vi "program.vi"() -> ()   [LabVIEW 2015]
panel:
  in  "Tab Control":enum32{"control", "diagnostics"}(tab)
  in  "Program":T1(array[cluster])=[{"Tstart"=95.0, "Tstop"=95.0, "rate(C/min)"=0.0, "time(min)"=5.0}, {"Tstart"=95.0, "Tstop"=90.0, "rate(C/min)"=240.0, "time(min)"=0.0}, {"Tstart"=90.0, "Tstop"=76.0, "rate(C/min)"=0.2, "time(min)"=0.0}, {"Tstart"=76.0, "Tstop"=26.0, "rate(C/min)"=0.067, "time(min)"=0.0}, {"Tstart"=25.0, "Tstop"=25.0, "rate(C/min)"=0.0, "time(min)"=30.0}] {"Tstop" min=20.0 max=100.0; "Tstart" min=20.0 max=100.0}
  out "XY Graph":cluster{dbl[], dbl[]}[](graph)
  out "temperature":dbl format="%.1f"
  in  "run":bool
  in  "abort":bool
  out "state":T2(ring)
  out "setpoint":dbl format="%.1f"
  in  "tolerance":dbl=1.0 format="%.2f"
  out "?":string
  out "concatenated string":string
  in  "dt(min)":dbl=1.0
  out "ptrace":cluster{dbl[], dbl[]}
  # "Instructions:  \n    1) Edit the program before starting the  VI\n    2) After starting, Hit Run or Abort as needed."
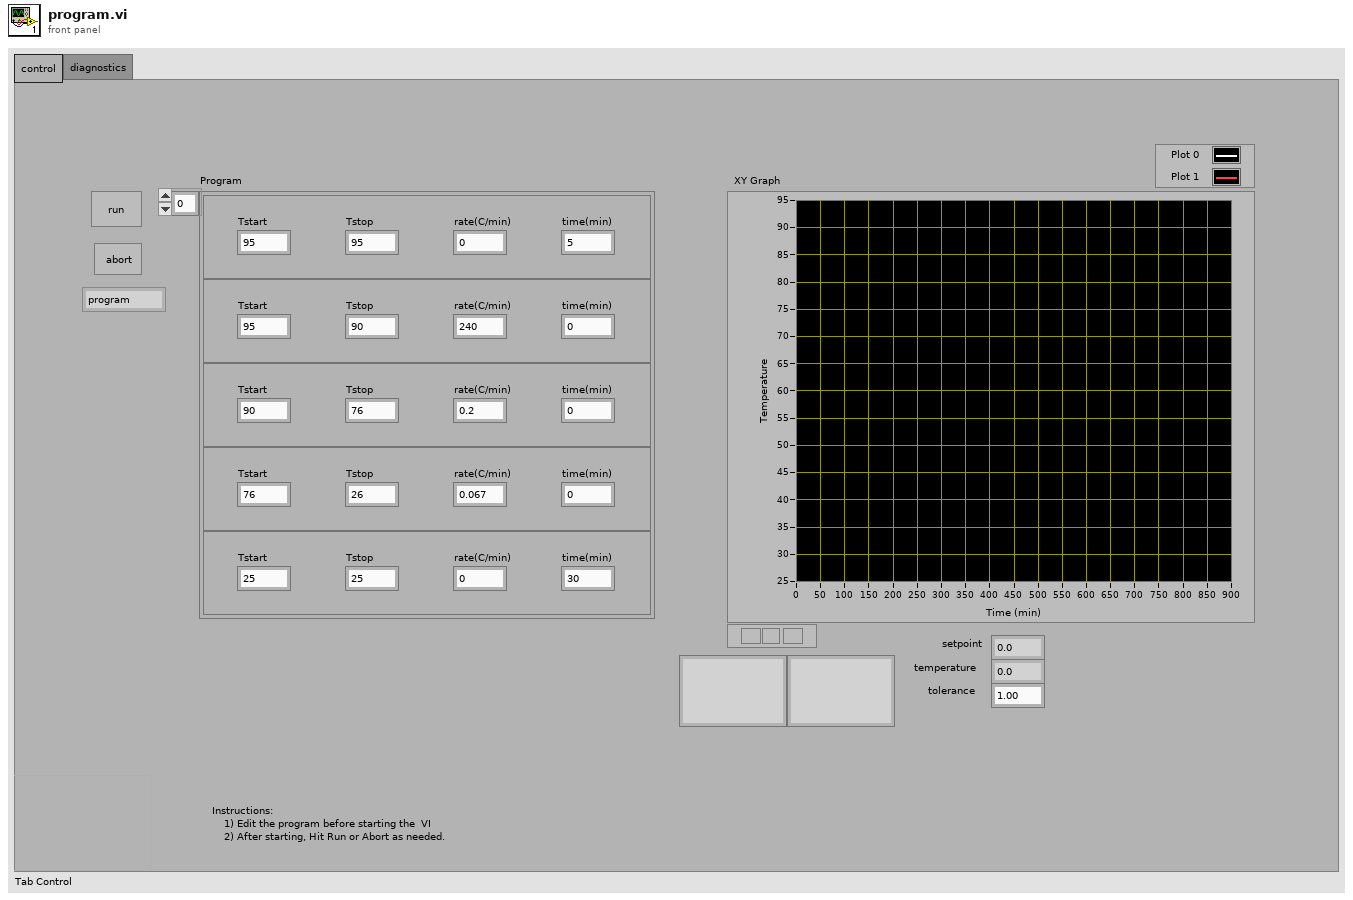
[diagram p1: front panel]
types:
  T1 = cluster{"Tstart":dbl, "Tstop":dbl, "rate(C/min)":dbl, "time(min)":dbl}[]
  T2 = enum16{"program", "init", "follow", "aborting", "quit"}
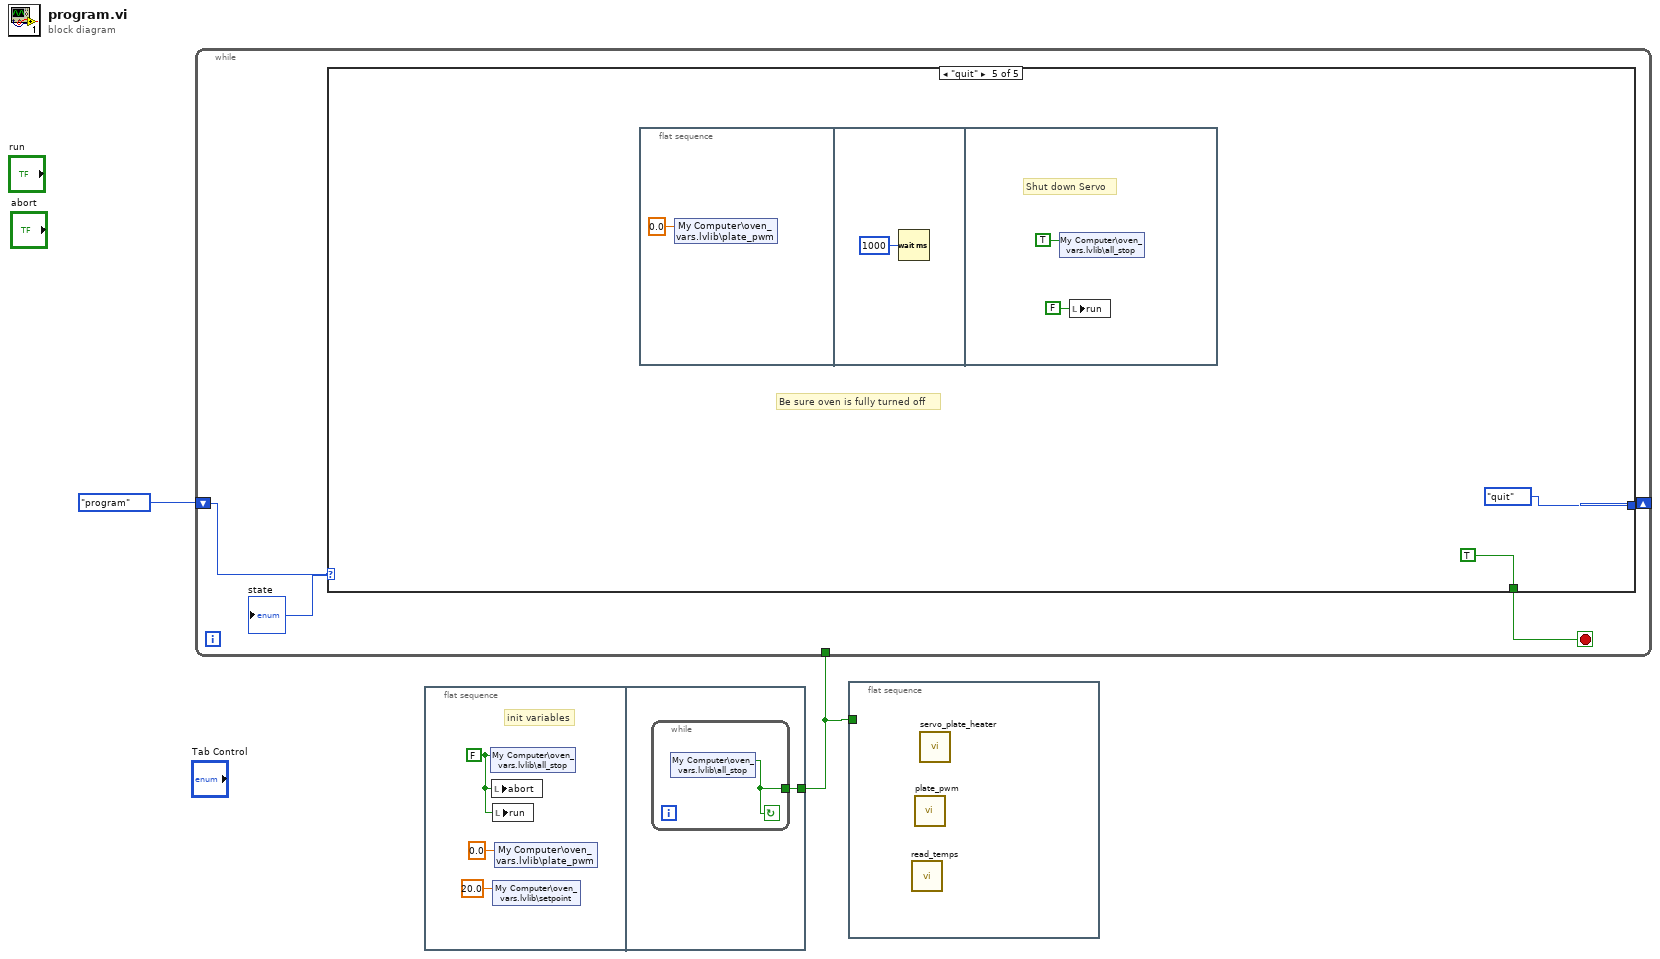
[diagram p0: block diagram]
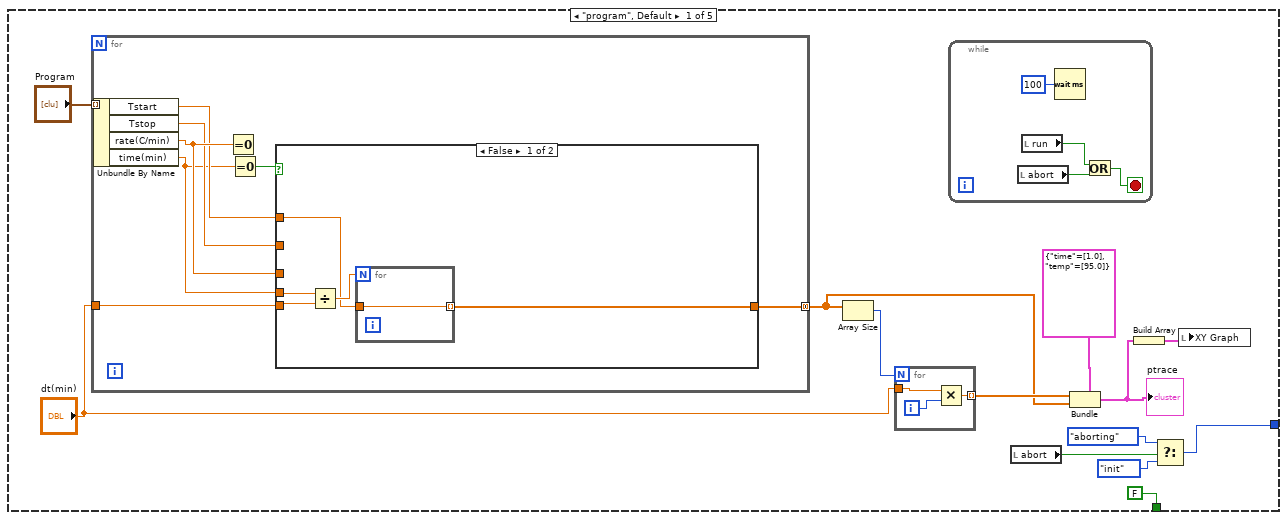
[diagram p2: hidden frame]
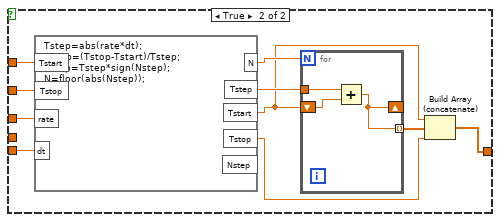
[diagram p3: hidden frame]
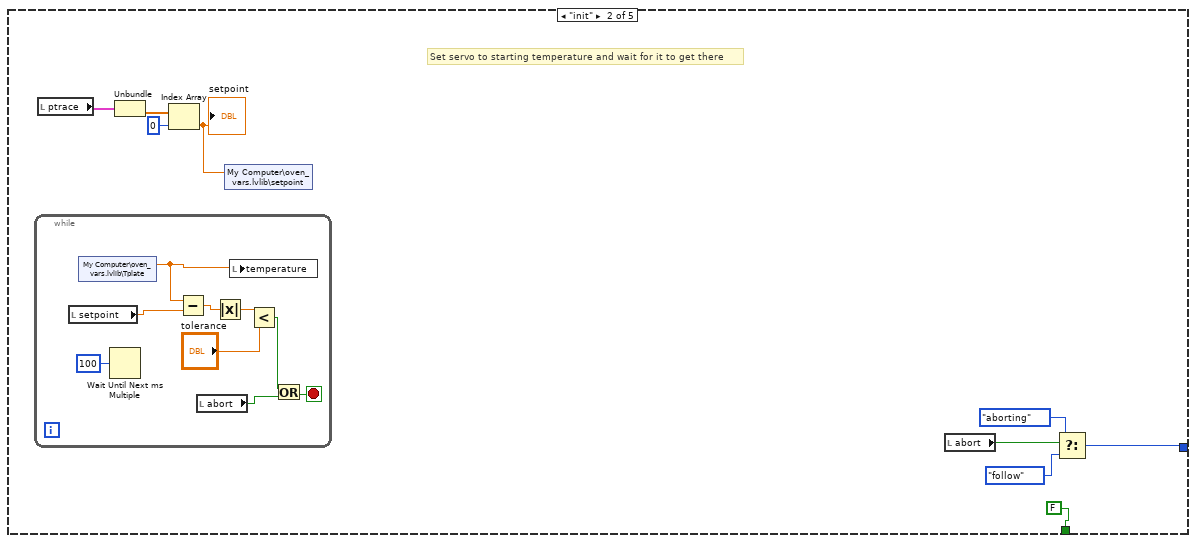
[diagram p4: hidden frame]
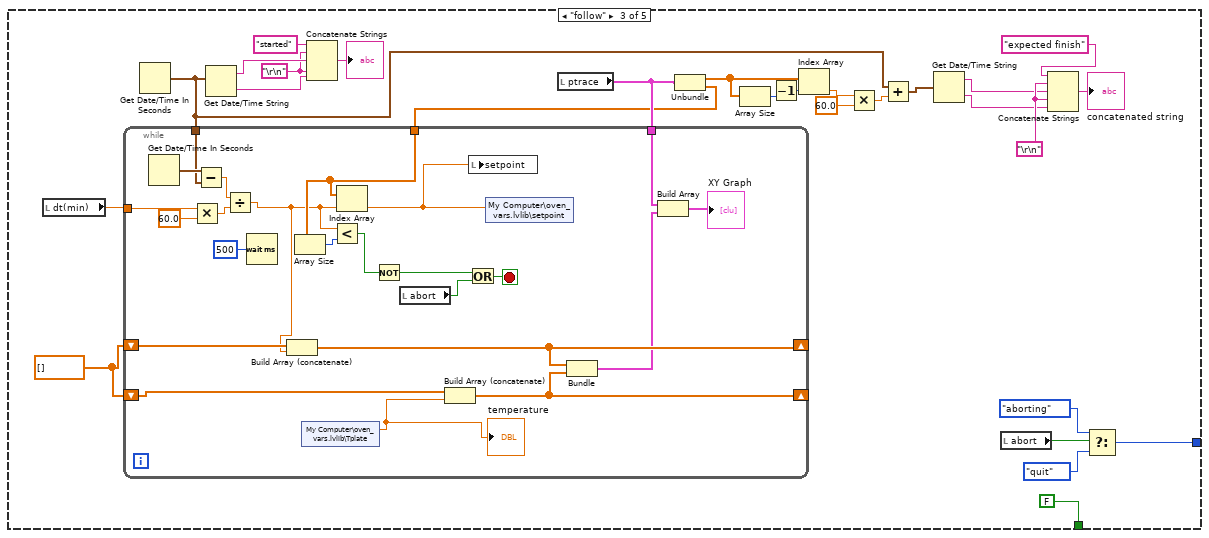
[diagram p5: hidden frame]
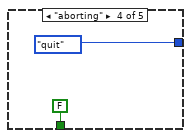
[diagram p6: hidden frame]
diagram:
  n1 = while {
    shift-right: [w5] -> _
    shift-left: T2."program" ("state") -> [w3]
    tunnel: w1 -> [_]
    stop <- w4 stop-if-true
    n2 = case shown="\"quit\"" w3 {
      tunnel: [w11 w57 w93 T2."quit" ("state") T2."quit" ("state")] -> w5
      tunnel: [FALSE FALSE FALSE FALSE TRUE] -> w4
      frame "program", Default {
        n3 = for {
          tunnel: "Program" -> [w33] mode=indexing
          tunnel: [w27] -> w14 mode=concatenating
          tunnel: "dt(min)" -> [w26]
          n4 = Unbundle By Name(w33) -> ("Tstart"=w31:dbl, "Tstop"=w30:dbl, "rate(C/min)"=w32:dbl, "time(min)"=w28:dbl)
          n5 = Equal To 0?(x=w32) -> ()  [unwired: 1 out]
          n6 = Equal To 0?(x=w28) -> (x = 0?=w29:bool)
          n7 = case shown="False" w29 {
            tunnel: w26 -> [w37 w49]
            tunnel: w32 -> [_ w48]
            tunnel: w31 -> [w35 w47]
            tunnel: w30 -> [_ w46]
            tunnel: w28 -> [w38 _]
            tunnel: [w34 w40] -> w27
            frame False {
              n8 = Divide(x=w38, y=w37) -> (x/y=w36:dbl)
              n9 = for {
                N: w36 -> [_]
                tunnel: w35 -> [w39]
                tunnel: [w39] -> w34 mode=indexing
              }
            }
            frame True {
              n10 = formula code="Tstep=abs(rate*dt);\nNstep=(Tstop-Tstart)/Tstep;\nTstep=Tstep*sign(Nstep);\nN=floor(abs(Nstep));"("Tstart"=w47, "Tstop"=w46, "rate"=w48, "dt"=w49) -> ("N"=w45:dbl, "Tstep"=w44:dbl, "Tstart"=w41:dbl, "Tstop"=w42:dbl)  [unwired: 1 out]
              n11 = for {
                N: w45 -> [_]
                shift-right: [w50] -> _
                shift-left: w41 -> [w52]
                tunnel: w44 -> [w51]
                tunnel: [w50] -> w43 mode=indexing
                n12 = Add(x=w51, y=w52) -> (x+y=w50:dbl)
              }
              n13 = Build Array (concatenate)(w41, w43, w42) -> (w40:dbl[])
            }
          }
        }
        n14 = Array Size(array=w14) -> (size(s)=w17:i32)
        n15 = for {
          N: w17 -> [_]
          tunnel: "dt(min)" -> [w24]
          tunnel: [w23] -> w16 mode=indexing
          i -> [w25]
          n16 = Multiply(x=w24, y=w25) -> (x*y=w23:dbl)
        }
        n17 = while {
          stop <- w22 stop-if-true
          n18 = local read "abort"() -> (w21:bool)
          n19 = local read "run"() -> (w20:bool)
          n20 = Wait (ms)(milliseconds to wait=u32 100) -> ()  [unwired: 1 out]
          n21 = Or(x=w20, y=w21) -> (x .or. y?=w22:bool)
        }
        n22 = local read "abort"() -> (w10:bool)
        n23 = Bundle(cluster=cluster{"time":dbl[], "temp":dbl[]} {"time"=[1.0], "temp"=[95.0]}, "time"=w16, "temp"=w14) -> (w6:cluster{"time":dbl[], "temp":dbl[]})
        "ptrace" <- w6
        n24 = Build Array(w6) -> (w7:cluster{"time":dbl[], "temp":dbl[]}[])
        n25 = Select(t=T2."aborting" ("state"), s=w10, f=T2."init" ("state")) -> (s? t:f=w11:T2)
        n26 = local write "XY Graph"(w7) -> ()
      }
      frame "init" {
        # "Set servo to starting temperature and wait for it to get there"
        n27 = while {
          stop <- w64 stop-if-true
          n28 = local read "setpoint"() -> (w70:dbl)
          n29 = shared-variable "My Computer\\oven_vars.lvlib\\Tplate"() -> (w62:dbl)  [unwired: 1 in, 1 out]
          n30 = Wait Until Next ms Multiple(millisecond multiple=u32 100) -> ()  [unwired: 1 out]
          n31 = Subtract(x=w62, y=w70) -> (x-y=w69:dbl)
          n32 = local read "abort"() -> (w63:bool)
          n33 = Absolute Value(x=w69) -> (abs(x)=w68:dbl)
          n34 = local write "temperature"(w62) -> ()
          n35 = Less?(x=w68, y="tolerance") -> (x < y?=w66:bool)
          n36 = Or(x=w66, y=w63) -> (x .or. y?=w64:bool)
        }
        n37 = local read "ptrace"() -> (w61:cluster{dbl[], dbl[]})
        n38 = Unbundle(w61) -> (w60:dbl[])  [unwired: 1 out]
        n39 = Index Array(array=w60, index=0) -> (element=w58:dbl)
        "setpoint" <- w58
        n40 = shared-variable "My Computer\\oven_vars.lvlib\\setpoint"(w58) -> ()  [unwired: 1 in, 1 out]
        n41 = local read "abort"() -> (w56:bool)
        n42 = Select(t=T2."aborting" ("state"), s=w56, f=T2."follow" ("state")) -> (s? t:f=w57:T2)
      }
      frame "follow" {
        w74 = "\r\n"
        w85 = "\r\n"
        w97 = dbl[] []
        n43 = local read "dt(min)"() -> (w94:dbl)
        n44 = Get Date/Time In Seconds() -> (seconds since 1Jan1904=w77:timestamp)
        n45 = Get Date/Time String(seconds (now)=w77) -> (date string=w87:string, time string=w86:string)  [unwired: 2 in]
        n46 = Concatenate Strings("started" ("string"), w85, w87, w85, w86) -> (→"?":string)
        n47 = local read "ptrace"() -> (w96:cluster{dbl[], dbl[]})
        n48 = Unbundle(w96) -> (w82:dbl[], w95:dbl[])
        n49 = while {
          tunnel: w77 -> [w119]
          tunnel: w94 -> [w115]
          tunnel: w95 -> [w104]
          shift-right: [w111] -> _
          shift-left: w97 -> [w113]
          shift-right: [w110] -> _
          shift-left: w97 -> [w112]
          tunnel: w96 -> [w108]
          stop <- w106 stop-if-true
          n50 = Get Date/Time In Seconds() -> (seconds since 1Jan1904=w120:timestamp)
          n51 = Multiply(x=w115, y=60.0) -> (x*y=w116:dbl)
          n52 = Subtract(x=w120, y=w119) -> (x-y=w117:dbl)
          n53 = Divide(x=w117, y=w116) -> (x/y=w102:dbl)
          n54 = Wait (ms)(milliseconds to wait=u32 500) -> ()  [unwired: 1 out]
          n55 = Build Array (concatenate)(w113, w102) -> (w111:dbl[])
          n56 = Array Size(array=w104) -> (size(s)=w103:i32)
          n57 = shared-variable "My Computer\\oven_vars.lvlib\\Tplate"() -> (w99:dbl)  [unwired: 1 in, 1 out]
          "temperature" <- w99
          n58 = Less?(x=w102, y=w103) -> (x < y?=w101:bool)
          n59 = Index Array(array=w104, index=w102) -> (element=w100:dbl)
          n60 = Not(x=w101) -> (.not. x?=w98:bool)
          n61 = local read "abort"() -> (w105:bool)
          n62 = Build Array (concatenate)(w112, w99) -> (w110:dbl[])
          n63 = Or(x=w98, y=w105) -> (x .or. y?=w106:bool)
          n64 = local write "setpoint"(w100) -> ()
          n65 = shared-variable "My Computer\\oven_vars.lvlib\\setpoint"(w100) -> ()  [unwired: 1 in, 1 out]
          n66 = Bundle(w111, w110) -> (w109:cluster{dbl[], dbl[]})  [unwired: 1 in]
          n67 = Build Array(w108, w109) -> (→"XY Graph":cluster{dbl[], dbl[]}[])
        }
        n68 = Array Size(array=w82) -> (size(s)=w83:i32)
        n69 = Decrement(x=w83) -> (x-1=w81:i32)
        n70 = Index Array(array=w82, index=w81) -> (element=w80:dbl)
        n71 = Multiply(x=w80, y=60.0) -> (x*y=w78:dbl)
        n72 = Add(x=w77, y=w78) -> (x+y=w76:timestamp)
        n73 = Get Date/Time String(seconds (now)=w76) -> (date string=w73:string, time string=w71:string)  [unwired: 2 in]
        n74 = local read "abort"() -> (w92:bool)
        n75 = Concatenate Strings("expected finish", w74, w73, w74, w71) -> (→"concatenated string":string)
        n76 = Select(t=T2."aborting" ("state"), s=w92, f=T2."quit" ("state")) -> (s? t:f=w93:T2)
      }
      frame "aborting" {
      }
      frame "quit" {
        # "Be sure oven is fully turned off"
        n77 = flat-sequence {
          frame #0 {
            n78 = shared-variable "My Computer\\oven_vars.lvlib\\plate_pwm"(0.0 ("plate_pwm")) -> ()  [unwired: 1 in, 1 out]
          }
          frame #1 {
            n79 = Wait (ms)(milliseconds to wait=u32 1000) -> ()  [unwired: 1 out]
          }
          frame #2 {
            # "Shut down Servo"
            n80 = shared-variable "My Computer\\oven_vars.lvlib\\all_stop"(TRUE ("all_stop")) -> ()  [unwired: 1 in, 1 out]
            n81 = local write "run"(FALSE ("run")) -> ()
          }
        }
      }
    }
    "state" <- w3
  }
  n82 = flat-sequence {
    tunnel: [w132] -> w1
    frame #0 {
      w129 = FALSE ("all_stop")
      # "init variables"
      n83 = shared-variable "My Computer\\oven_vars.lvlib\\all_stop"(w129) -> ()  [unwired: 1 in, 1 out]
      n84 = local write "abort"(w129) -> ()
      n85 = local write "run"(w129) -> ()
      n86 = shared-variable "My Computer\\oven_vars.lvlib\\setpoint"(20.0 ("setpoint")) -> ()  [unwired: 1 in, 1 out]
      n87 = shared-variable "My Computer\\oven_vars.lvlib\\plate_pwm"(0.0 ("plate_pwm")) -> ()  [unwired: 1 in, 1 out]
    }
    frame #1 {
      n88 = while {
        tunnel: [w133] -> w132
        stop <- w133 continue-if-true
        n89 = shared-variable "My Computer\\oven_vars.lvlib\\all_stop"() -> (w133:bool)  [unwired: 1 in, 1 out]
      }
    }
  }
  n90 = flat-sequence {
    tunnel: w1 -> [_]
    frame #0 {
      n91 = call "read_temps.vi"() -> ()  [unwired: 12 in]
      n92 = call "plate_pwm.vi"() -> ()  [unwired: 12 in]
      n93 = call "servo_plate_heater.vi"() -> ()  [unwired: 12 in]
    }
  }
